vi "verify related shutter parameters.vi"(8 "error in (no error)":errorcluster, 11 "Simulated_CCD_Camera in":refnum<class "Sim_Ixon_Ultra.lvclass">) -> (0 "error out":errorcluster, 3 "Simulated_CCD_Camera out":refnum<class "Sim_Ixon_Ultra.lvclass">)   [LabVIEW 2018, in "Sim_Ixon_Ultra.lvclass"]
doc: "Verify the related parameters of the camera\n\nThere are some parameters of the camera operation mode that depend on the value provided for another parameter. This function verifies if these parameters are in agreement."
uses:
  Sim_Ixon_Ultra.lvclass
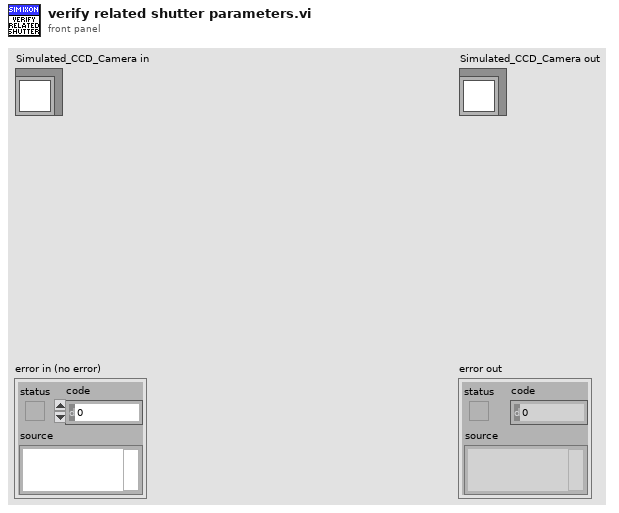
[diagram p1: front panel]
types:
  T1 = cluster{"PREAMP":u16, "READOUT_RATE":u16, "EM_GAIN":u16, "VERTICAL_SHIFT_SPEED":u16, "READ_MODE":u16, "FRAME_TRANSFER":bool, "VERTICAL_CLOCK_VOLTAGE":u16, "ACQUISITION_MODE":u16, "AD_CHANNEL":u16, "EM_MODE":u16, "SHUTTER_TTL":u16, "SHUTTER_OPENING_TIME":u16, "SHUTTER_CLOSING_TIME":u16, "SHUTTER_MODE":u16, "TRIGGER_MODE":u16, "VBIN":u16, "INITIAL_LINE":u16, "INITIAL_COLUMN":u16, "FINAL_LINE":u16, "FINAL_COLUMN":u16, "HBIN":u16}
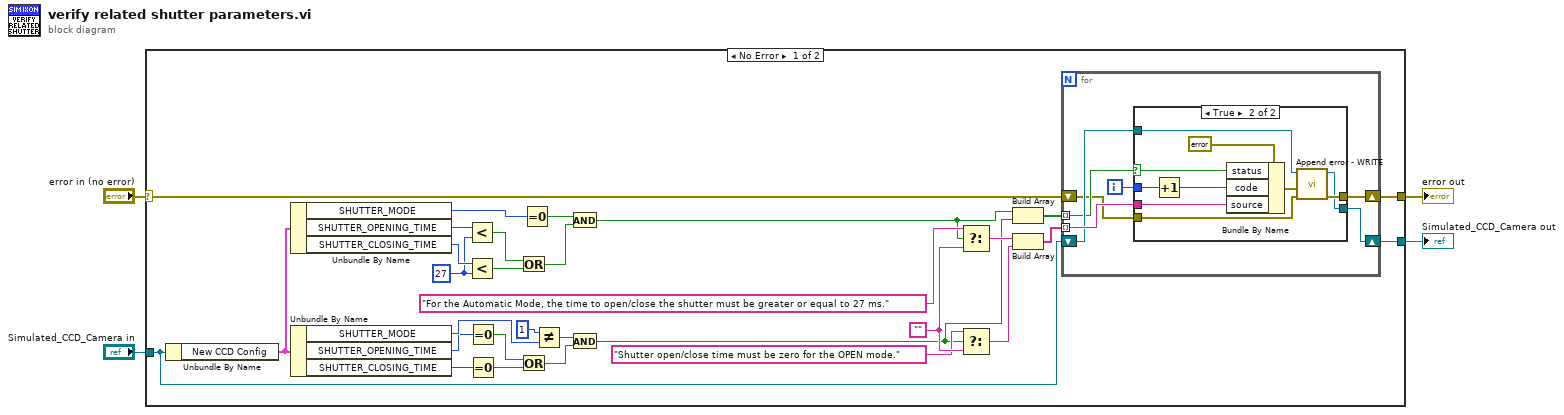
[diagram p0: block diagram]
diagram:
  n1 = case shown="No Error" "error in (no error)" {
    selector: "error in (no error)" -> [w7 w55]
    tunnel: [w6 w55] -> w3
    tunnel: [w8 w54] -> w1
    tunnel: "Simulated_CCD_Camera in" -> [w5 w54]
    frame No Error {
      w27 = 27
      w14 = ""
      n2 = Unbundle By Name(w5) -> ("New CCD Config"=w10:T1)
      n3 = Unbundle By Name(w10) -> ("SHUTTER_MODE"=w31:u16, "SHUTTER_OPENING_TIME"=w29:u16, "SHUTTER_CLOSING_TIME"=w28:u16)
      n4 = Unbundle By Name(w10) -> ("SHUTTER_MODE"=w22:u16, "SHUTTER_OPENING_TIME"=w20:u16, "SHUTTER_CLOSING_TIME"=w19:u16)
      n5 = Less?(x=w29, y=w27) -> (x < y?=w26:bool)
      n6 = Less?(x=w28, y=w27) -> (x < y?=w25:bool)
      n7 = Equal To 0?(x=w20) -> (x = 0?=w18:bool)
      n8 = Equal To 0?(x=w19) -> (x = 0?=w17:bool)
      n9 = Or(x=w26, y=w25) -> (x .or. y?=w24:bool)
      n10 = Or(x=w18, y=w17) -> (x .or. y?=w16:bool)
      n11 = Equal To 0?(x=w31) -> (x = 0?=w30:bool)
      n12 = Not Equal?(x=u16 1, y=w22) -> (x != y?=w15:bool)
      n13 = And(x=w30, y=w24) -> (x .and. y?=w23:bool)
      n14 = And(x=w15, y=w16) -> (x .and. y?=w12:bool)
      n15 = Select(t="For the Automatic Mode, the time to open/close the shutter must be greater or equal to 27 ms.", s=w23, f=w14) -> (s? t:f=w33:string)
      n16 = Select(t="Shutter open/close time must be zero for the OPEN mode.", s=w12, f=w14) -> (s? t:f=w11:string)
      n17 = Build Array(w23, w12) -> (w9:bool[])
      n18 = Build Array(w33, w11) -> (w34:string[])
      n19 = for {
        tunnel: w34 -> [w41] mode=indexing
        tunnel: w9 -> [w37] mode=indexing
        shift-right: [w38] -> w8
        shift-left: w5 -> [w39]
        shift-right: [w35] -> w6
        shift-left: w7 -> [w36]
        i -> [w40]
        n20 = case shown="True" w37 {
          selector: w37 -> [_ w49]
          tunnel: w41 -> [_ w53]
          tunnel: w40 -> [_ w52]
          tunnel: w39 -> [w43 w45]
          tunnel: [w43 w46] -> w38
          tunnel: w36 -> [w42 w48]
          tunnel: [w42 w47] -> w35
          frame False {
          }
          frame True {
            n21 = Increment(x=w52) -> (x+1=w51:i32)
            n22 = Bundle By Name(cluster=errorcluster {"status"=FALSE, "code"=0, "source"=""} ("error constant"), "status"=w49, "code"=w51, "source"=w53) -> (w44:errorcluster)
            n23 = call "Append error - WRITE.vi"("error in (no error)"=w48, "error"=w44, "Simulated_CCD_Camera in"=w45) -> ("error out"=w47:errorcluster, "Simulated_CCD_Camera out"=w46:refnum<class "Sim_Ixon_Ultra.lvclass">)  [unwired: 7 in]
          }
        }
      }
    }
    frame Error {
    }
  }
  "error out" <- w3
  "Simulated_CCD_Camera out" <- w1
